vi "App_Logout.vi"(8 "error in":errorcluster) -> (0 "error out":errorcluster)   [LabVIEW 2015, in "Application 2.lvlib"]
uses:
  Application 2.lvlib
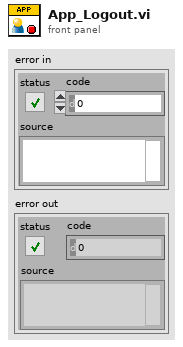
[diagram p1: front panel]
types:
  T1 = typedef "Application 2.lvlib/App_Main Data.ctl" = cluster{"VI Refnum":refnum<vi>, "Subpanel":refnum<vi>, "Connection ID":refnum<k5>, "Meta data":T2[], "Main Queue":T4, "User Data":T5}
  T2 = typedef "stm_MetaElement.ctl" = cluster{"Name":T3}
  T3 = typedef "stm_MetaDataElement.ctl" = string
  T4 = typedef "Application 2.lvlib/App_Main Queue.ctl" = cluster{"Main Loop Queue":refnum<queue>}
  T5 = typedef "User Data.ctl" = cluster{"Name":string, "Email":string, "Phone Number":string, "User Picture":u32[][], "Last Login Time":timestamp}
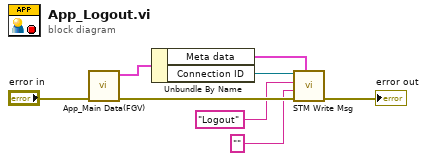
[diagram p0: block diagram]
diagram:
  n1 = call "App_Main Data(FGV).vi"("error in"="error in") -> ("error out"=w6:errorcluster, "Main Data Out"=w7:T1)  [unwired: 9 in]
  n2 = Unbundle By Name(w7) -> ("Meta data"=w5:T2[], "Connection ID"=w4:refnum<k5>)
  n3 = call "STM Write Msg.vi"("Meta data"=w5, "error in (no error)"=w6, "Data"="", "Name"="Logout", "connection ID"=w4) -> ("error out"=→"error out":errorcluster)  [unwired: 5 in, 1 out]
